vi "Launch Sub Loop.vi"(9 "Subscription Info":T2, 10 "Subscription":T1, 11 "ChannelService":refnum<class "ChannelService.lvclass">) -> (0 "error out":errorcluster)   [LabVIEW 2020, in "Vecto.lvlib" / "RemoteDataService.lvclass"]
uses:
  RemoteDataService.lvclass
  Subscription Info.ctl
  Subscription.ctl
  ChannelService/ChannelService.lvclass
  Subscription Loop.vi
  RemoteDataService.lvclass/RemoteDataService.ctl
  lv-promises/Promises/Promise/Promise.lvclass
  lv-promises/Promises/Error Result/Error Result.lvclass
  C:/dev/lv20CE/relink/lv-promises/Promises/Value/Value.lvclass
  C:/dev/lv20CE/relink/lv-promises/Promises/Error Result/Error Result.lvclass
  lv-promises/Promises/Future/Future.lvclass
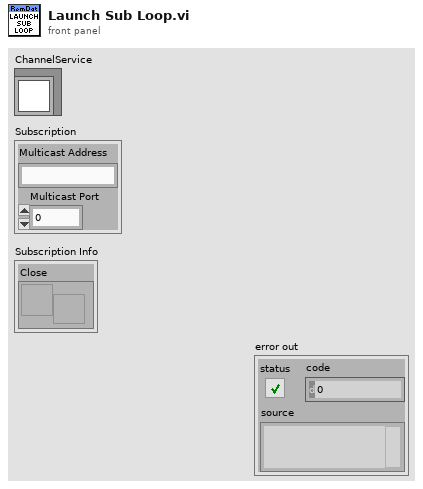
[diagram p1: front panel]
types:
  T1 = typedef "Vecto.lvlib/RemoteDataService.lvclass/Subscription.ctl" = cluster{"Multicast Address":string, "Multicast Port":u16}
  T2 = typedef "Vecto.lvlib/RemoteDataService.lvclass/Subscription Info.ctl" = cluster{"Close":refnum<user-event>}
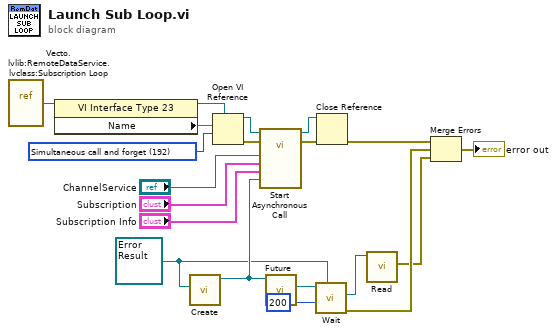
[diagram p0: block diagram]
diagram:
  w7 = refnum<class "Error Result.lvclass"> refnum ("Futures:Error Result.lvclass")
  w15 = 192 items=["Record modifications"=1, "Open templates for editing"=2, "Prompt user to save"=4, "Prepare for reentrant run"=8, "Prompt to find missing subVIs"=16, "Hide loading dialog box"=32, "Enable simultaneous calls"=64, "Prepare to call and forget"=128, "Simultaneous call and forget"=192, "Prepare to call and collect"=256, "Simultaneous call and collect"=320]
  n1 = vi-ref "Vecto.lvlib:RemoteDataService.lvclass:Subscription Loop.vi"() -> (w13:refnum<vi>)
  n2 = property class="VI Interface Type 23"(reference=w13) -> (reference out=w16:refnum<vi>, "Name"=w14:string)  [unwired: 1 in, 1 out]
  n3 = call "Create.vi"("Result Type"=w7) -> ("Promise"=w9:refnum<class "Promise.lvclass">)  [unwired: 9 in, 1 out]
  n4 = Open VI Reference(type specifier VI Refnum (for type only)=w16, vi path=w14, options=w15) -> (vi reference=w18:refnum<vi>, error out=w17:errorcluster)  [unwired: 3 in]
  n5 = call-by-ref "Start Asynchronous Call"(reference=w18, error in=w17, "Init Promise"=w9, "Subscription Info"="Subscription Info", "Subscription"="Subscription", "ChannelService"="ChannelService") -> (reference out=w20:refnum<vi>, error out=w19:errorcluster)  [unwired: 8 in]
  n6 = call "Future.vi"("Promise in"=w9) -> ("Future"=w8:refnum<class "Future.lvclass">)  [unwired: 9 in, 1 out]
  n7 = call "Wait.vi"("Result Type"=w7, "Timeout mS (-1)"=200, "Future in"=w8) -> ("error out"=w3:errorcluster, "Result"=w6:refnum<class "Error Result.lvclass">)  [unwired: 7 in]
  n8 = Close Reference(reference=w20, error in (no error)=w19) -> (error out=w5:errorcluster)
  n9 = call "Read.vi"("Error Result in"=w6) -> ("Error"=w2:errorcluster)  [unwired: 10 in]
  n10 = Merge Errors(w5, w3, w2) -> (→"error out":errorcluster)
